vi "test-unscented-kalman-filter-2.vi"() -> (3 "Test good":bool)   [LabVIEW 2019]
uses:
  <vilib>/Analysis/Matrix/Datatypes/RealMatrix.ctl
  <vilib>/Rock Robotics/WPI/ThirdParty/JAS_Junk/TrajLib/UNSCENTED_KALMAN_FILTER.ctl
  <vilib>/Rock Robotics/WPI/ThirdParty/JAS_Junk/TrajLib/MERWE_SCALED_SIGMA_PTS.ctl
  <vilib>/Rock Robotics/WPI/ThirdParty/JAS_Junk/TrajLib/CALLBACK_FUNC_TYPE.ctl
  <vilib>/Analysis/baseanly.llb/Real A x B.vi
  <vilib>/Rock Robotics/WPI/ThirdParty/JAS_Junk/TrajLib/MatBuilder_Create.vi
  <vilib>/Rock Robotics/WPI/ThirdParty/JAS_Junk/TrajLib/LinearSystem_New.vi
  <vilib>/Rock Robotics/WPI/ThirdParty/JAS_Junk/TrajLib/MatrixHelper_Zero.vi
  <vilib>/Rock Robotics/WPI/ThirdParty/JAS_Junk/TrajLib/MatBuilder_Fill.vi
  <vilib>/Rock Robotics/WPI/ThirdParty/JAS_Junk/TrajLib/MatrixHelper_CoerceSize.vi
  <vilib>/Rock Robotics/WPI/ThirdParty/JAS_Junk/TrajLib/Matrix_Exp.vi
  <vilib>/Rock Robotics/WPI/ThirdParty/JAS_Junk/TrajLib/Matrix_AssignBlock.vi
  <vilib>/Rock Robotics/WPI/ThirdParty/JAS_Junk/TrajLib/Matrix_ExtractFrom.vi
  <vilib>/Analysis/7linalg.llb/Matrix Exp.vi
  <vilib>/Analysis/7linalg.llb/Real Matrix Exp.vi
  <vilib>/Analysis/Matrix/Numeric/Multiply/Multiply.vi
  <vilib>/Analysis/Matrix/Numeric/Multiply/Multiply - RM,R.vi
  <vilib>/Analysis/Matrix/Numeric/Subtract/Subtract - RM,RM.vi
  <vilib>/Analysis/7linalg.llb/Solve Linear Equations (multiple right hand).vi
  <vilib>/Rock Robotics/WPI/ThirdParty/JAS_Junk/TrajLib/Trajectory_Library.lvlib
  <vilib>/Analysis/NI_AALPro.lvlib
  <vilib>/Analysis/NI_AALBase.lvlib
  <vilib>/Analysis/Matrix/NI_Matrix.lvlib
panel:
  out "Ref Value":dbl
  out "out UnscentedKalmanFiilter":T1
  out "xHat":T2
  out "Error 00":errorcluster
  # "State Estimate <Statess,1>"
  # "<States, States>"
  # "<States, ?>"
  # "<Statess,  States>"
  # "<Outputs, Outputs>"
  # "<?, 1>"
  # "<?, 1>"
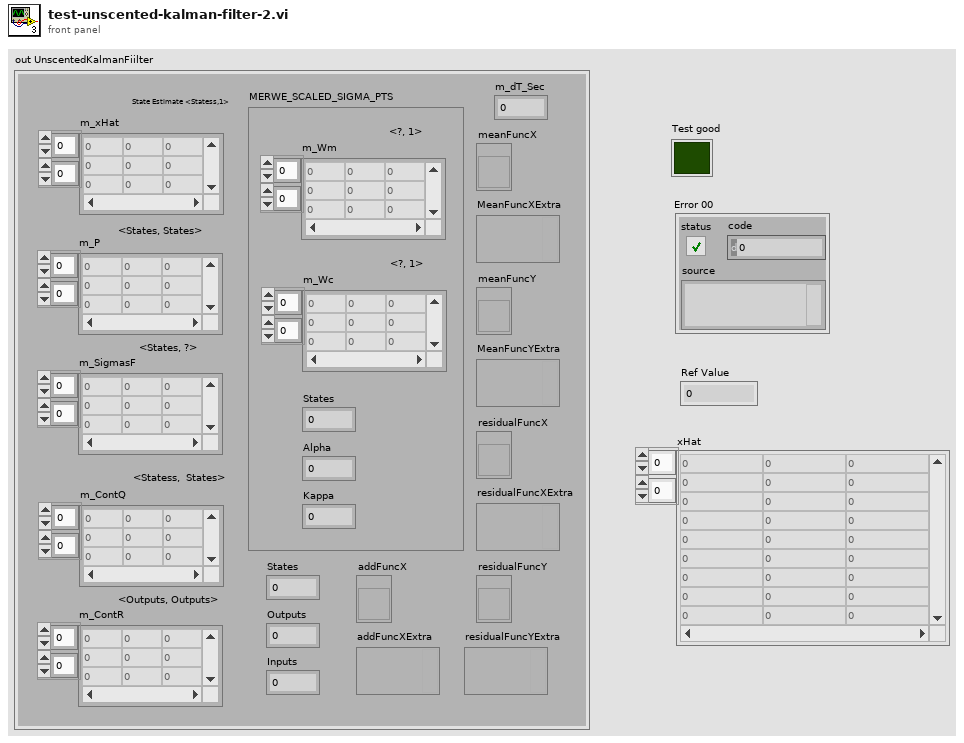
[diagram p1: front panel]
types:
  T1 = typedef "Trajectory_Library.lvlib/UNSCENTED_KALMAN_FILTER.ctl" = cluster{"m_P":T2, "m_xHat":T2, "States":i32, "Outputs":i32, "m_ContR":T2, "m_ContQ":T2, "m_SigmasF":T2, "m_dT_Sec":dbl, "MERWE_SCALED_SIGMA_PTS":T3, "meanFuncX":T4, "meanFuncY":T4, "residualFuncX":T4, "residualFuncY":T4, "addFuncX":T4, "addFuncXExtra":variant, "residualFuncYExtra":variant, "residualFuncXExtra":variant, "MeanFuncYExtra":variant, "MeanFuncXExtra":variant, "Inputs":i32}
  T2 = typedef "NI_Matrix.lvlib/RealMatrix.ctl" = dbl[][]
  T3 = typedef "Trajectory_Library.lvlib/MERWE_SCALED_SIGMA_PTS.ctl" = cluster{"m_Wm":T2, "States":i32, "Alpha":dbl, "m_Wc":T2, "Kappa":i32}
  T4 = typedef "Trajectory_Library.lvlib/CALLBACK_FUNC_TYPE.ctl" = refnum<vi>
  T5 = typedef "Trajectory_Library.lvlib/LINEAR_SYSTEM.ctl" = cluster{"m_A":T2, "m_B":T2, "m_C":T2, "m_D":T2, "States":i32, "Inputs":i32, "Outputs":i32}
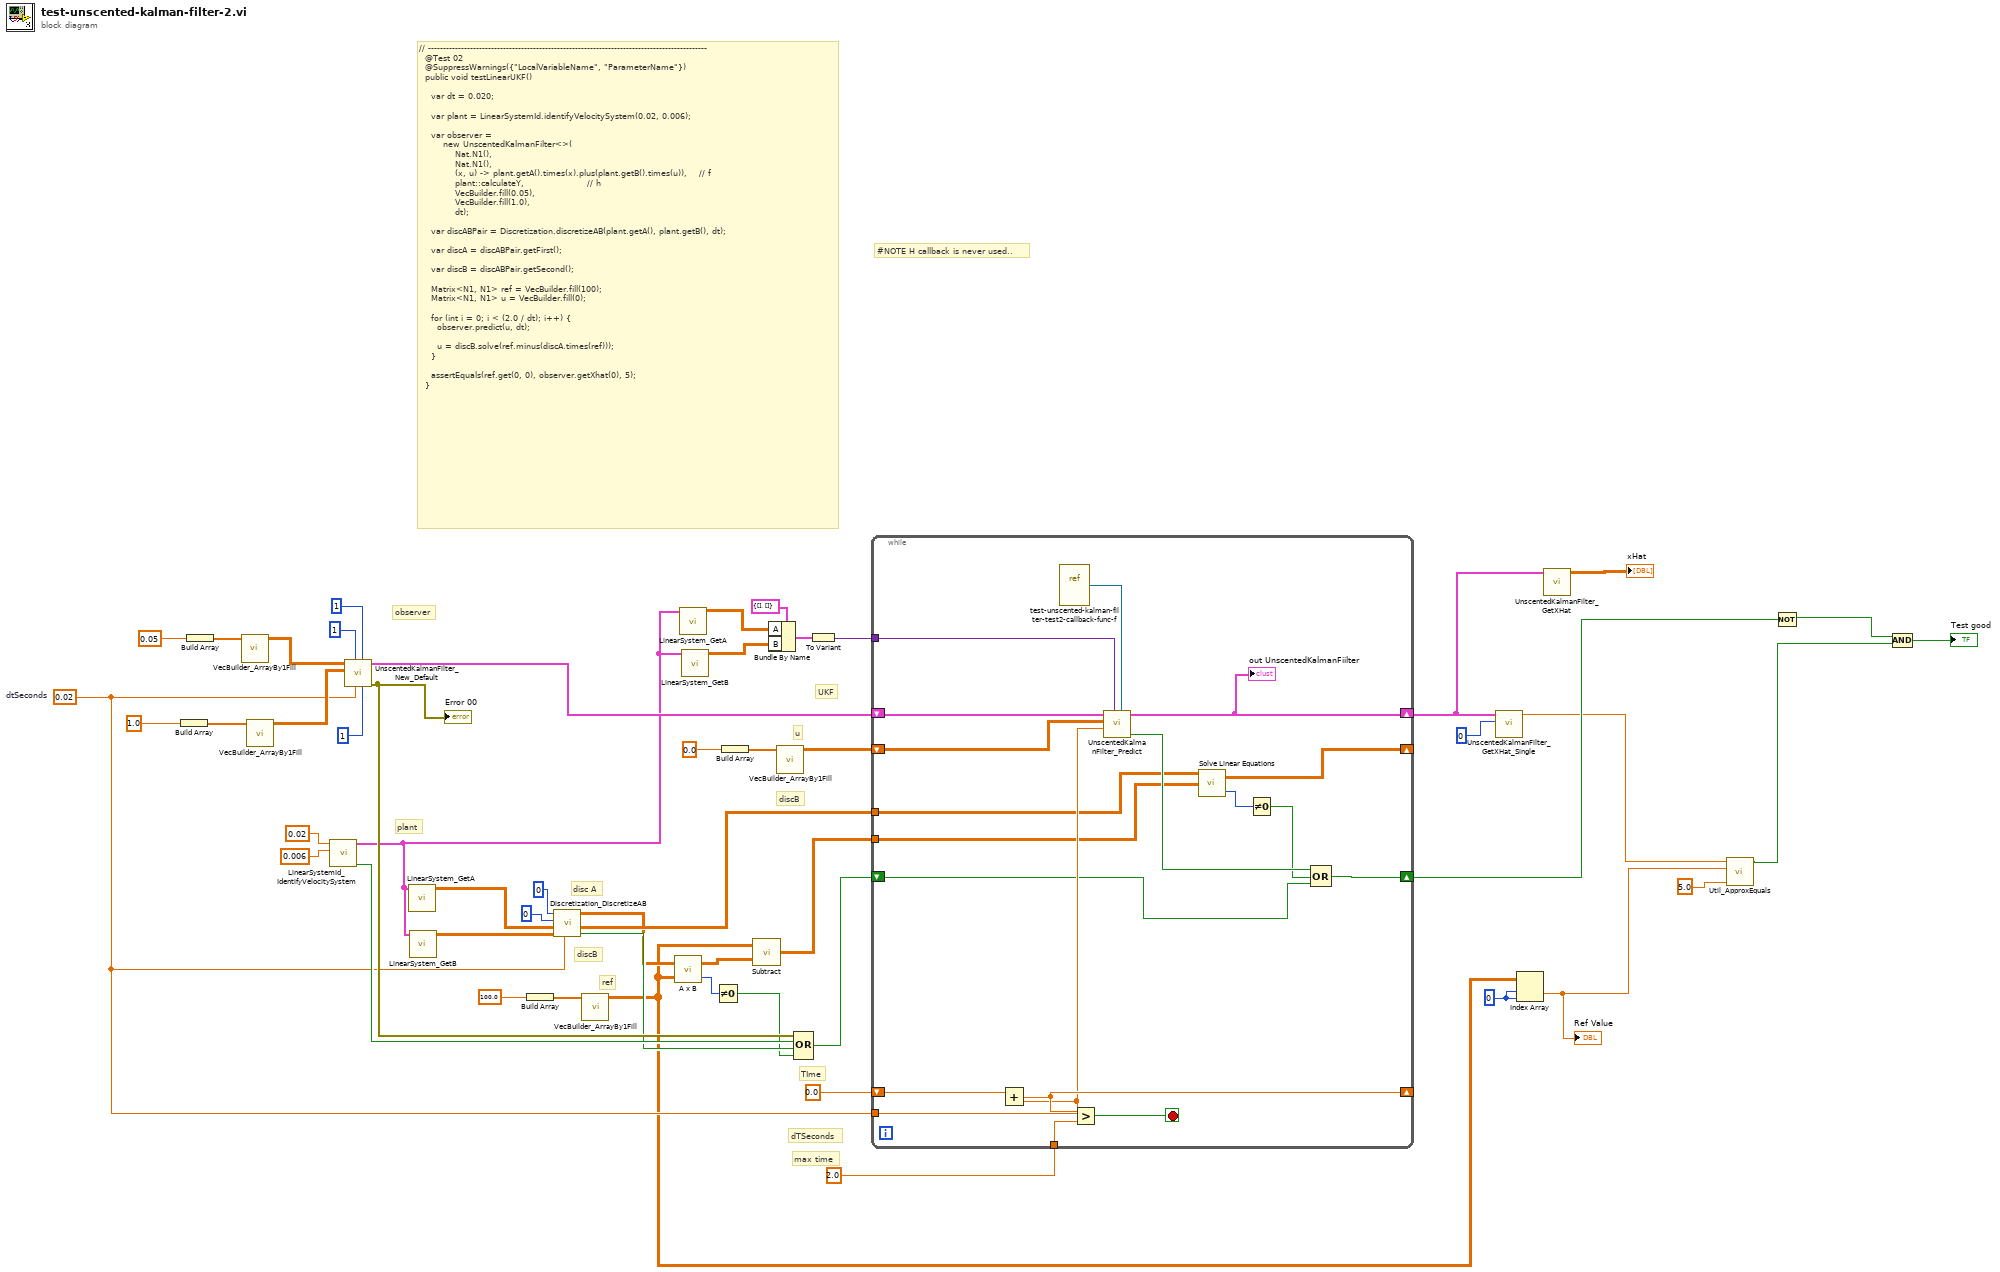
[diagram p0: block diagram]
diagram:
  w9 = 0 ("index (row)")
  w28 = 0.02  # dtSeconds
  # "UKF"
  # "#NOTE H callback is never used.."
  # "discB"
  # "max time"
  # "u"
  # "ref"
  # "discB"
  # "disc A"
  # "observer"
  # "plant"
  # "// ---------------------------------------------------------------------------------------------\n  @Test 02\n  @SuppressWarnings({\"LocalVariableName\", \"ParameterName\"})\n  public void testLinearUKF() \n\n    var dt = 0.020;\n\n    var plant = LinearSystemId.identifyVelocitySystem(0.02, 0.006);\n\n    var observer =\n        new UnscentedKalmanFilter<>(\n            Nat.N1(),\n            Nat.N1(),\n            (x, u) -> plant.getA().times(x).plus(plant.getB().times(u)),    // f\n            plant::calculateY,                     // h\n            VecBuilder.fill(0.05),\n            VecBuilder.fill(1.0),\n            dt);\n\n    var discABPair = Discretization.discretizeAB(plant.getA(), plant.getB(), dt);\n\n    var discA = discABPair.getFirst();\n\n    var discB = discABPair.getSecond();\n\n    Matrix<N1, N1> ref = VecBuilder.fill(100);\n    Matrix<N1, N1> u = VecBuilder.fill(0);\n\n    for (int i = 0; i < (2.0 / dt); i++) {\n      observer.predict(u, dt);\n\n      u = discB.solve(ref.minus(discA.times(ref)));\n    }\n\n    assertEquals(ref.get(0, 0), observer.getXhat(0), 5);\n  }"
  # "dTSeconds"
  # "TIme"
  n1 = Build Array(1.0 ("element")) -> (w46:dbl[])
  n2 = Build Array(0.05 ("element")) -> (w49:dbl[])
  n3 = call <vilib>:"VecBuilder_ArrayBy1Fill.vi"("R Array"=w49) -> ("Output Vector"=w44:T2)  [unwired: 10 in]
  n4 = call <vilib>:"VecBuilder_ArrayBy1Fill.vi"("R Array"=w46) -> ("Output Vector"=w45:T2)  [unwired: 10 in]
  n5 = call <vilib>:"LinearSystemId_IdentifyVelocitySystem.vi"("kA"=0.006, "kV"=0.02) -> ("Size Coerced"=w33:bool, "Linearsystem"=w6:T5)  [unwired: 8 in]
  n6 = call <vilib>:"UnscentedKalmanFilter_New_Default.vi"("Inputs"=1, "States"=1, "dt_Seconds"=w28, "Outputs"=1, "MeasurementStdDevs"=w45, "StateStdDevs"=w44) -> ("Error"=w37:errorcluster, "UnscentedKalmanFiilter"=w21:T1)  [unwired: 4 in]
  "Error 00" <- w37
  n7 = call <vilib>:"LinearSystem_GetA.vi"("Linearsystem"=w6) -> ("A"=w30:T2)  [unwired: 10 in]
  n8 = call <vilib>:"LinearSystem_GetB.vi"("Linearsystem"=w6) -> ("B"=w29:T2)  [unwired: 10 in]
  n9 = Build Array(100.0 ("element")) -> (w26:dbl[])
  n10 = call <vilib>:"Discretization_DiscretizeAB.vi"("dT_Seconds"=w28, "ContB"=w29, "ContA"=w30, "Inputs"=0, "States"=0) -> ("Error"=w27:bool, "DiscB"=w19:T2, "DiscA"=w18:T2)  [unwired: 4 in]
  n11 = call <vilib>:"VecBuilder_ArrayBy1Fill.vi"("R Array"=w26) -> ("Output Vector"=w10:T2)  [unwired: 10 in]
  n12 = call-poly <vilib>:"A x B.vi"("B"=w10, "A"=w18) -> ("error"=w15:i32, "A x B"=w17:T2)
  n13 = call <vilib>:"LinearSystem_GetA.vi"("Linearsystem"=w6) -> ("A"=w4:T2)  [unwired: 10 in]
  n14 = call <vilib>:"LinearSystem_GetB.vi"("Linearsystem"=w6) -> ("B"=w5:T2)  [unwired: 10 in]
  n15 = Not Equal To 0?(x=w15) -> (x != 0?=w14:bool)
  n16 = Build Array(0.0 ("element")) -> (w24:dbl[])
  n17 = call-poly <vilib>:"Subtract.vi"("Real Matrix B"=w17, "Real Matrix A"=w10) -> ("A - B"=w16:T2)
  n18 = Bundle By Name(cluster=cluster{"A":T2, "B":T2} {"A"=[], "B"=[]} ("Cluster"), "A"=w4, "B"=w5) -> (w3:cluster{"A":T2, "B":T2})
  n19 = call <vilib>:"VecBuilder_ArrayBy1Fill.vi"("R Array"=w24) -> ("Output Vector"=w20:T2)  [unwired: 10 in]
  n20 = Compound Arithmetic op=OR(w37, w33, w27, w14) -> (w38:bool)
  n21 = To Variant(anything=w3) -> (Variant=w1:variant)
  n22 = while {
    shift-right: [w68] -> _
    shift-left: 0.0 -> [w70]
    tunnel: w28 -> [w63]
    shift-right: [w67] -> w12
    shift-left: w38 -> [w55]
    tunnel: 2.0 -> [w66]
    shift-right: [w61] -> w11
    shift-left: w21 -> [w65]
    shift-right: [w58] -> _
    shift-left: w20 -> [w64]
    tunnel: w19 -> [w60]
    tunnel: w16 -> [w59]
    tunnel: w1 -> [w53]
    stop <- w69 stop-if-true
    n23 = Add(x=w70, y=w63) -> (x+y=w68:dbl)
    n24 = vi-ref "test-unscented-kalman-filter-test2-callback-func-f.vi"() -> (w54:refnum<vi>)
    n25 = Greater?(x=w68, y=w66) -> (0:w69:bool)
    n26 = call <vilib>:"UnscentedKalmanFilter_Predict.vi"("f_Func"=w54, "F_Func_ExtraData"=w53, "dT_Seconds"=w63, "U"=w64, "in UnscentedKalmanFiilter"=w65) -> ("Error"=w62:bool, "out UnscentedKalmanFiilter"=w61:T1)  [unwired: 5 in]
    "out UnscentedKalmanFiilter" <- w61
    n27 = call-poly <vilib>:"Solve Linear Equations.vi"("Known Matrix"=w59, "Input Matrix"=w60) -> ("error"=w57:i32, "Solution Matrix"=w58:T2)  [unwired: 1 in]
    n28 = Not Equal To 0?(x=w57) -> (x != 0?=w56:bool)
    n29 = Compound Arithmetic op=OR(w62, w56, w55) -> (w67:bool)
  }
  n30 = call <vilib>:"UnscentedKalmanFilter_GetXHat_Single.vi"("Row"=0, "in UnscentedKalmanFiilter"=w11) -> ("xHat Value"=w8:dbl)  [unwired: 9 in]
  n31 = Index Array(array=w10, index (row)=w9, index (col)=w9) -> (element=w7:dbl)
  "Ref Value" <- w7
  n32 = call <vilib>:"UnscentedKalmanFilter_GetXHat.vi"("in UnscentedKalmanFiilter"=w11) -> ("xHat"=→"xHat":T2)  [unwired: 10 in]
  n33 = call <vilib>:"Util_ApproxEquals.vi"("Tolerance"=5.0, "Value 2"=w7, "Value 1"=w8) -> ("ApproxEquals"=w36:bool)  [unwired: 8 in]
  n34 = Not(x=w12) -> (.not. x?=w39:bool)
  n35 = Compound Arithmetic op=AND(w39, w36) -> (→"Test good":bool)
